vi "F_a_4.vi"() -> ()   [LabVIEW 2014]
uses:
  <vilib>/Analysis/baseanly.llb/Real Dot Product.vi
  <vilib>/Analysis/2dsp.llb/Real FFT.vi
  <vilib>/Analysis/NI_AALBase.lvlib
  <vilib>/Analysis/NI_AALPro.lvlib
panel:
  out "Waveform Graph":dbl[](graph)
  out "Señal de entrada y Salida":dbl[](graph)
  out "o_e":dbl[](array[numeric])
  out "o_s":dbl[](array[numeric])
  in  "beta":dbl
  out "delay":dbl[](array[numeric])
  out "w":dbl[](array[numeric])
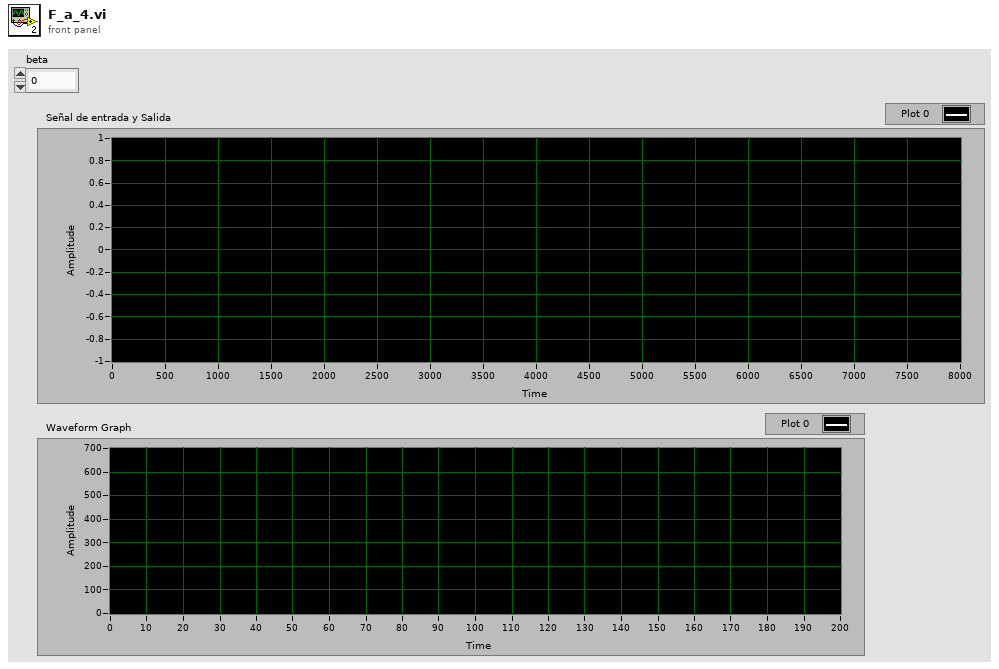
[diagram p1: front panel]
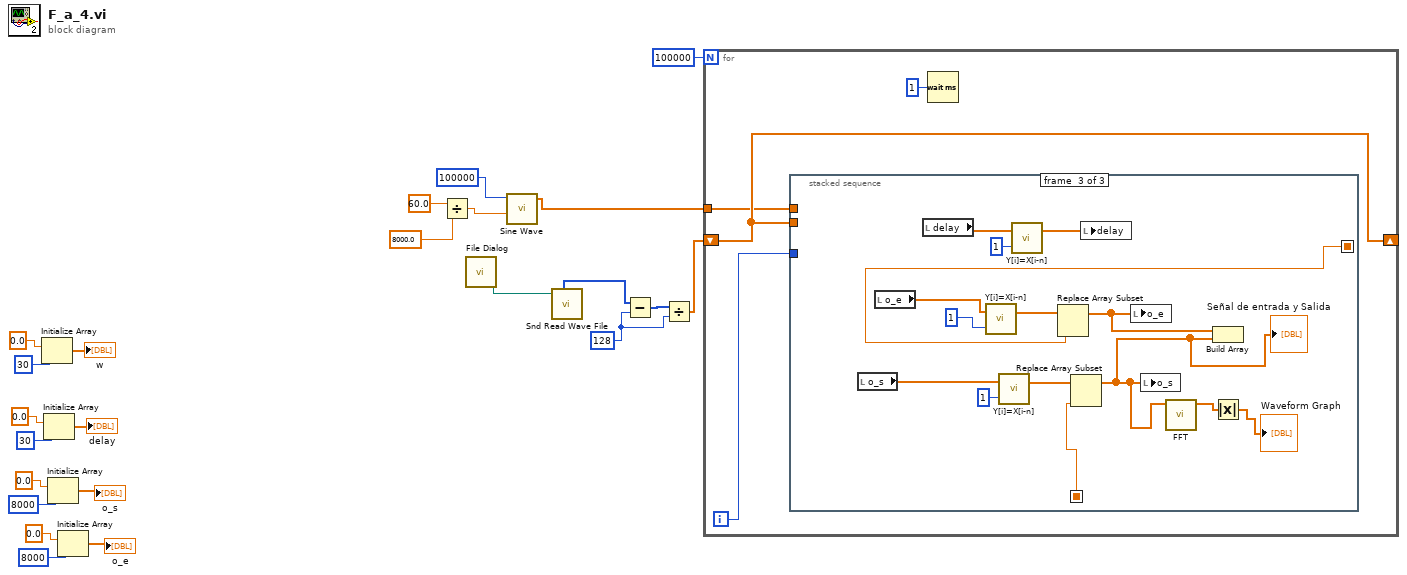
[diagram p0: block diagram]
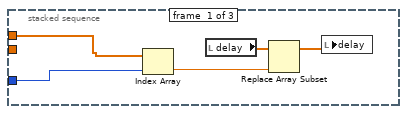
[diagram p2: hidden frame]
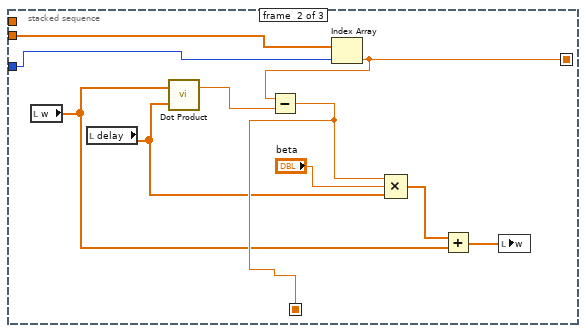
[diagram p3: hidden frame]
diagram:
  w6 = 128
  n1 = Initialize Array(0.0 ("element"), 30 ("dimension size")) -> (→"w":dbl[])
  n2 = Initialize Array(0.0 ("element"), 30 ("dimension size")) -> (→"delay":dbl[])
  n3 = Initialize Array(0.0 ("element"), 8000 ("dimension size")) -> (→"o_s":dbl[])
  n4 = Initialize Array(0.0 ("element"), 8000 ("dimension size")) -> (→"o_e":dbl[])
  n5 = Divide(x=60.0, y=8000.0) -> (x/y=w21:dbl)
  n6 = call "File Dialog"() -> ("selected path"=w23:path)  [unwired: 12 in, 3 out]
  n7 = call <vilib>:"Sine Wave.vi"("samples"=100000, "frequency"=w21) -> ("sine wave"=w1:dbl[])  [unwired: 3 in, 2 out]
  n8 = call "Snd Read Wave File.vi"("wave file path"=w23) -> ("mono 8-bit"=w8:u8[])  [unwired: 4 in, 6 out]
  n9 = Subtract(x=w8, y=w6) -> (x-y=w7:i32[])
  n10 = Divide(x=w7, y=w6) -> (x/y=w5:dbl[])
  n11 = for {
    N: 100000 -> [_]
    shift-right: [w26] -> _
    shift-left: w5 -> [w26]
    tunnel: w1 -> [w25]
    i -> [w27]
    n12 = stacked-sequence {
      seq-local: [_ w39 _] -> [_ _ w51]
      seq-local: [_ w35 _] -> [_ _ w46]
      tunnel: w27 -> [w31 w42 _]
      tunnel: w26 -> [_ w38 _]
      tunnel: w25 -> [w30 _ _]
      frame #0 {
        n13 = Index Array(array=w30, index=w31) -> (element=w28:dbl)
        n14 = local read "delay"() -> (w32:dbl[])
        n15 = Replace Array Subset(array=w32, new element=w28) -> (w29:dbl[])  [unwired: 1 in]
        n16 = local write "delay"(w29) -> ()
      }
      frame #1 {
        n17 = local read "w"() -> (w33:dbl[])
        n18 = local read "delay"() -> (w34:dbl[])
        n19 = call-poly <vilib>:"Dot Product.vi"("Y Vector"=w34, "X Vector"=w33) -> ("X * Y"=w40:dbl)  [unwired: 1 out]
        n20 = Index Array(array=w38, index=w42) -> (element=w35:dbl)
        n21 = Subtract(x=w35, y=w40) -> (x-y=w39:dbl)
        n22 = Compound Arithmetic op=MULTIPLY(w39, "beta", w34) -> (w36:dbl[])
        n23 = Add(x=w36, y=w33) -> (x+y=w37:dbl[])
        n24 = local write "w"(w37) -> ()
      }
      frame #2 {
        n25 = local read "o_s"() -> (w54:dbl[])
        n26 = local read "o_e"() -> (w48:dbl[])
        n27 = local read "delay"() -> (w57:dbl[])
        n28 = call <vilib>:"Y[i]=X[i-n].vi"("shifts: n"=1, "Input Array"=w48) -> ("Shifted Array"=w49:dbl[])  [unwired: 1 out]
        n29 = call <vilib>:"Y[i]=X[i-n].vi"("shifts: n"=1, "Input Array"=w54) -> ("Shifted Array"=w52:dbl[])  [unwired: 1 out]
        n30 = call <vilib>:"Y[i]=X[i-n].vi"("shifts: n"=1, "Input Array"=w57) -> ("Shifted Array"=w55:dbl[])  [unwired: 1 out]
        n31 = Replace Array Subset(array=w49, new element=w46) -> (w47:dbl[])  [unwired: 1 in]
        n32 = Replace Array Subset(array=w52, new element=w51) -> (w44:dbl[])  [unwired: 1 in]
        "Señal de entrada y Salida" <- w44
        n33 = local write "delay"(w55) -> ()
        n34 = local write "o_e"(w47) -> ()
        n35 = local write "o_s"(w44) -> ()
        n36 = call-poly <vilib>:"FFT.vi"("X"=w44) -> ("FFT {X}"=w45:cdb[])  [unwired: 9 in, 1 out]
        n37 = Build Array(w47, w44) -> ()  [unwired: 1 out]
        n38 = Absolute Value(x=w45) -> (abs(x)=→"Waveform Graph":dbl[])
      }
    }
    n39 = Wait (ms)(milliseconds to wait=u32 1) -> ()  [unwired: 1 out]
  }
